vi "AssertsVIExecState.vi"(11 "error in":errorcluster) -> (15 "error out":errorcluster)   [LabVIEW 2016, in "DronaTest.lvlib"]
uses:
  DronaTest.lvlib
  APIs/Assert/AssertVI/AssertVIExecNotBad.vi
  APIs/Assert/AssertVI/AssertVIExecRunning.vi
  APIs/Stimulus/VI/CloseVI.vi
  APIs/Assert/AssertVI/AssertVIExecIdle.vi
  <vilib>/addons/_JKI Toolkits/Caraya/classes/Test/Test.lvclass
  Drona.lvlib
  APIs/Stimulus/VI/VI.lvlib
  APIs/Assert/AssertVI/AssertVI.lvlib
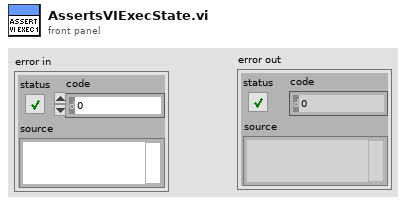
[diagram p1: front panel]
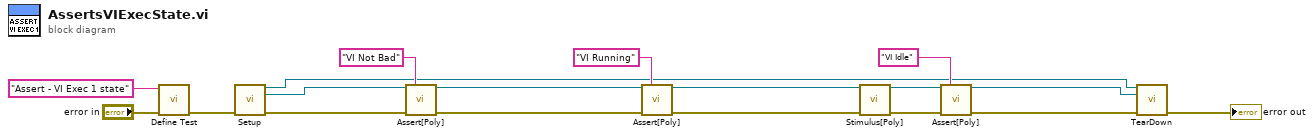
[diagram p0: block diagram]
diagram:
  n1 = call <vilib>:"Define Test.vi"("error in (no error)"="error in", "Label (VI Title)"="Assert - VI Exec 1 state" ("string")) -> ("error out"=w14:errorcluster)  [unwired: 9 in]
  n2 = call "Setup.vi"("error in (no error)"=w14) -> ("Application Ref"=w2:refnum<vi>, "VI out"=w7:refnum<vi>, "error out"=w8:errorcluster)  [unwired: 12 in]
  n3 = call-poly "Assert[Poly].vi"("VI Reference In"=w7, "Test Label"="VI Not Bad" ("Label"), "Error In"=w8) -> ("VI Reference Out"=w5:refnum<vi>, "Error Out"=w6:errorcluster)  [unwired: 11 in]
  n4 = call-poly "Assert[Poly].vi"("VI Reference In"=w5, "Test Label"="VI Running" ("Label"), "Error In"=w6) -> ("VI Reference Out"=w3:refnum<vi>, "Error Out"=w4:errorcluster)  [unwired: 11 in]
  n5 = call-poly "Stimulus[Poly].vi"("VI Reference In"=w3, "error in"=w4) -> ("VI Reference Out"=w12:refnum<vi>, "error out"=w13:errorcluster)  [unwired: 12 in]
  n6 = call-poly "Assert[Poly].vi"("VI Reference In"=w12, "Test Label"="VI Idle" ("Label"), "Error In"=w13) -> ("VI Reference Out"=w9:refnum<vi>, "Error Out"=w10:errorcluster)  [unwired: 11 in]
  n7 = call "TearDown.vi"("Application Ref"=w2, "VI in"=w9, "error in (no error)"=w10) -> ("error out"=→"error out":errorcluster)  [unwired: 12 in]
